vi "add glyphs from path.vi"(8 "error in (no error)":errorcluster, 10 "Path":path, 11 "glyph manager in":T1) -> (0 "error out":errorcluster, 3 "glyph manager out":T1)   [LabVIEW 2023, in "CEF.lvlib"]
doc: "Copyright 2017 National Instruments Corporation\n\nLicensed under the Apache License, Version 2.0 (the \"License\"); you may not use this file except in compliance with the License. You may obtain a copy of the License at http://www.apache.org/licenses/LICENSE-2.0\nUnless required by applicable law or agreed to in writing, software distributed under the License is distributed on an \"AS IS\" BASIS, WITHOUT WARRANTIES OR CONDITIONS OF ANY KIND, either express or implied. See the License for the specific language governing permissions and limitations under the License."
uses:
  CEF.lvlib
  glyph manager.ctl
  <vilib>/picture/picture.llb/imagedata.ctl
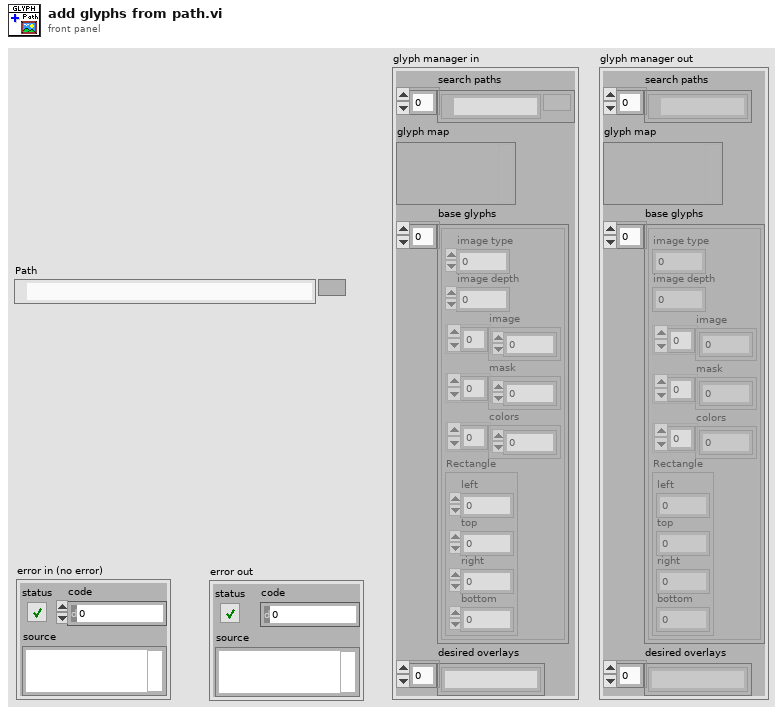
[diagram p1: front panel]
types:
  T1 = typedef "CEF.lvlib/glyph manager.ctl" = cluster{"search paths":path[], "glyph map":variant, "base glyphs":T2[], "desired overlays":string[]}
  T2 = typedef "imagedata.ctl" = cluster{"image type":i32, "image depth":i32, "image":u8[], "mask":u8[], "colors":u32[], "Rectangle":cluster{"left":i16, "top":i16, "right":i16, "bottom":i16}}
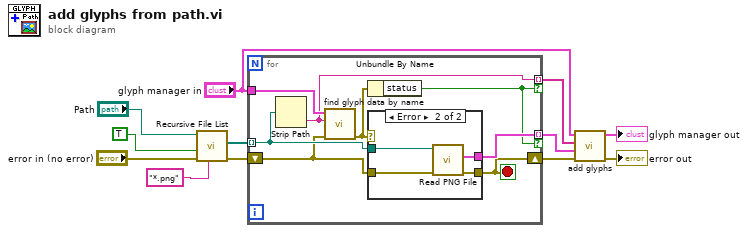
[diagram p0: block diagram]
diagram:
  n1 = call <vilib>:"Recursive File List.vi"("pattern"="*.png", "error in (no error)"="error in (no error)", "Continue Recursing on Error? (F)"=TRUE, "Folder Path"="Path") -> ("error out"=w10:errorcluster, "All Files in Dir"=w9:path[])  [unwired: 3 in, 3 out]
  n2 = for {
    tunnel: w9 -> [w20] mode=indexing
    shift-right: [w13] -> w11
    shift-left: w10 -> [w14]
    tunnel: [w19] -> w2 mode=indexing if=w16
    tunnel: [w15] -> w3 mode=indexing if=w16
    tunnel: "glyph manager in" -> [w18]
    stop <- w13 stop-if-true
    n3 = Strip Path(path=w20) -> (name=w15:string)  [unwired: 1 out]
    n4 = call "find glyph data by name.vi"("error in"=w14, "name"=w15, "glyph manager in"=w18) -> ("error out"=w17:errorcluster)  [unwired: 5 in, 3 out]
    n5 = Unbundle By Name(w17) -> ("status"=w16:bool)
    n6 = case shown="Error" w17 {
      tunnel: [w21 w23] -> w13
      tunnel: w14 -> [w21 w24]
      tunnel: w20 -> [_ w25]
      tunnel: [_ w22] -> w19
      frame No Error {
      }
      frame Error {
        n7 = call <vilib>:"Read PNG File.vi"("error in (no error)"=w24, "path to PNG file"=w25) -> ("error out"=w23:errorcluster, "image data"=w22:T2)  [unwired: 7 in, 1 out]
      }
    }
  }
  n8 = call "add glyphs.vi"("error in"=w11, "glyphs"=w2, "names"=w3, "glyph manager in"="glyph manager in") -> ("error out"=→"error out":errorcluster, "glyph manager out"=→"glyph manager out":T1)  [unwired: 6 in]
